vi "Data File Processing UI Default Runtime Menu Path.vi"() -> (8 "runtime menu path":path)   [LabVIEW 2012]
panel:
  # "Input Data"
  # "Local Data"
  # "Output Data"
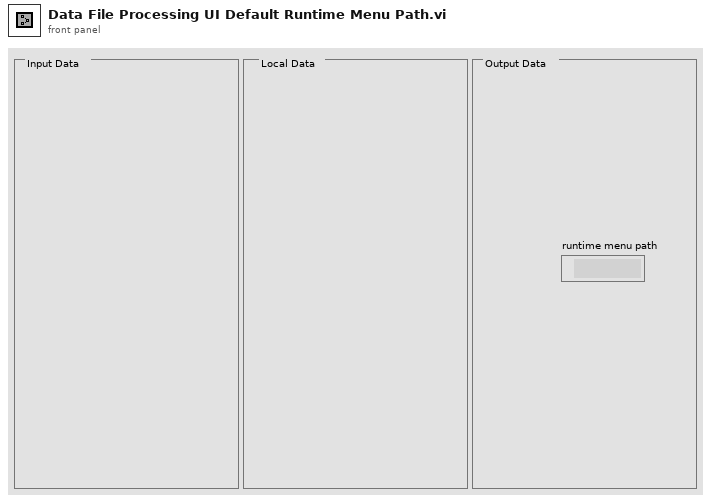
[diagram p1: front panel]
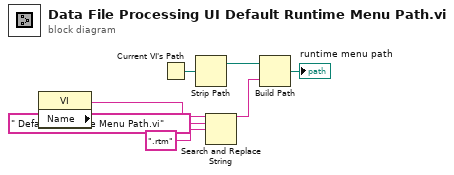
[diagram p0: block diagram]
diagram:
  n1 = property class="VI"() -> ("Name"=w6:string)  [unwired: 2 in, 2 out]
  n2 = Current VI's Path() -> (path=w7:path)
  n3 = Strip Path(path=w7) -> (stripped path=w2:path)  [unwired: 1 out]
  n4 = Search and Replace String(input string=w6, search string=" Default Runtime Menu Path.vi", replace string=".rtm" ("replace string (\"\")")) -> (result string=w3:string)  [unwired: 5 in, 3 out]
  n5 = Build Path(base path=w2, name or relative path=w3) -> (appended path=→"runtime menu path":path)
